vi "H3C psw cable 28G SFP+读写操作_old.vi"(6 "input_psw":u8[](array[numeric]) format="%.0x", 8 "input_data":u8[](array[numeric]) format="%.0x", 9 "input_mode":string(combo), 10 "Channel":u8 max=5 step=1, 11 "VISA":refnum<visa-resource-name>="COM6") -> (0 "A2Hequal00?":bool, 1 "result":bool, 2 "message":string, 3 "data read":u8[](array[numeric]) format="%.0x")   [LabVIEW 2011]
panel:
  out "A2h后128个字节":u8[](array[numeric]) format="%.0x"
  out "A2h前128个字节":u8[](array[numeric]) format="%.0x"
  in  "address":u8
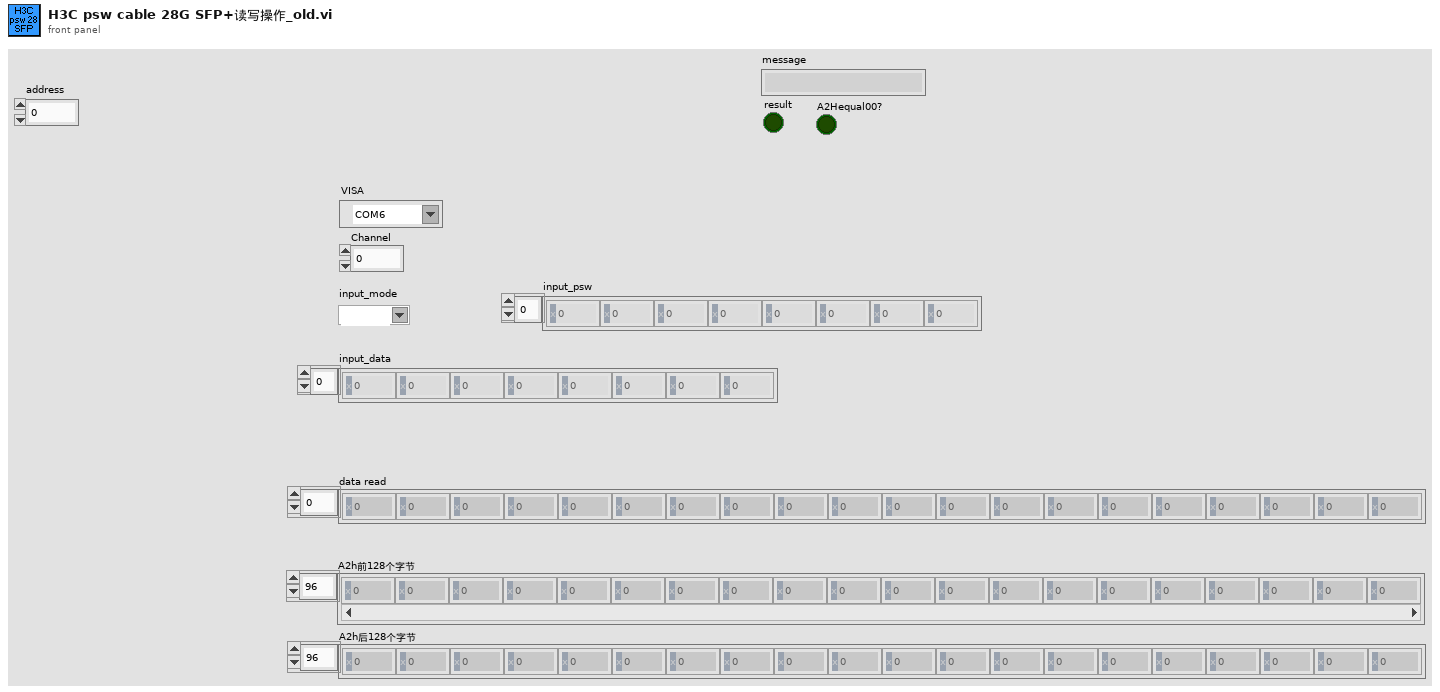
[diagram p1: front panel]
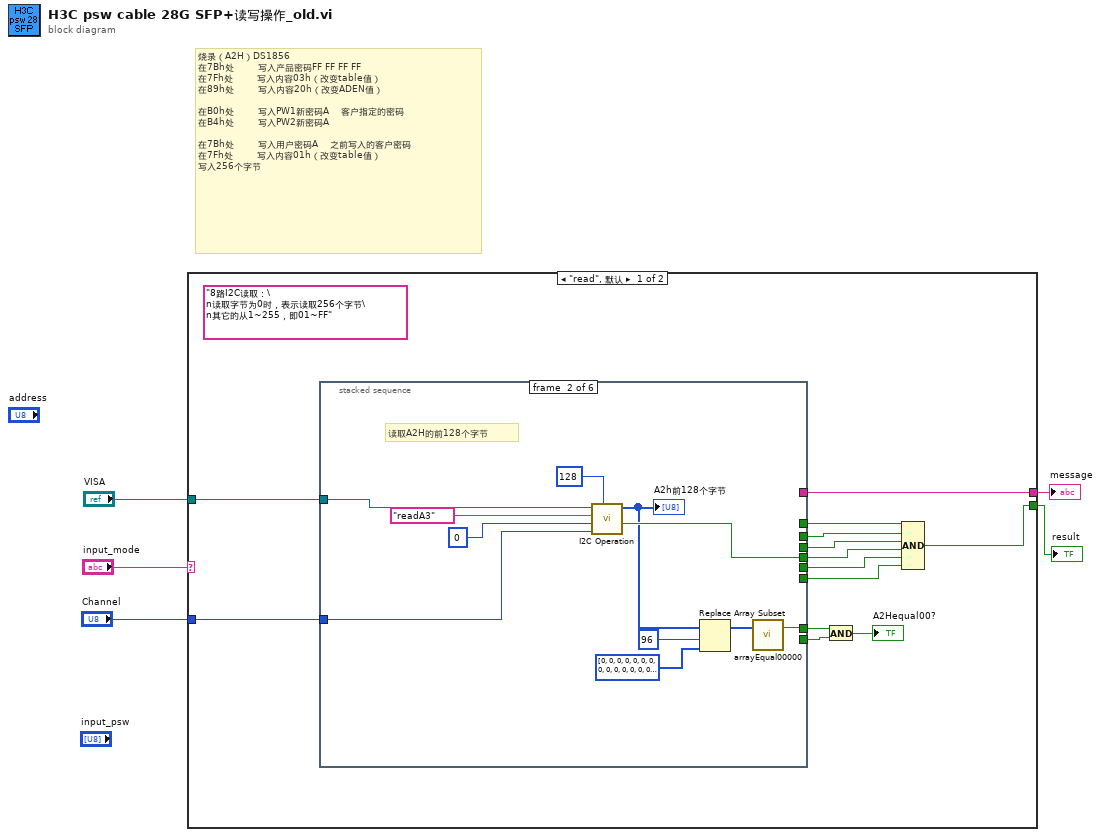
[diagram p0: block diagram]
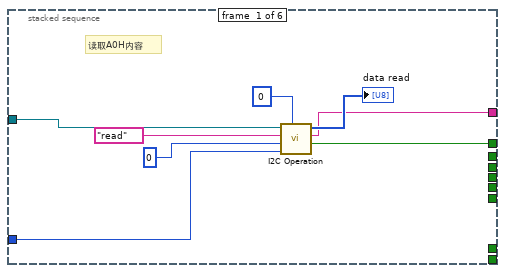
[diagram p2: hidden frame]
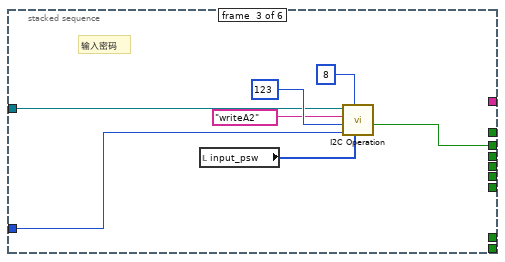
[diagram p3: hidden frame]
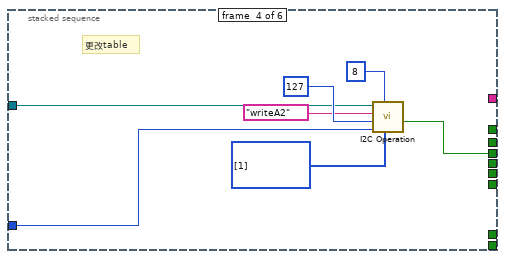
[diagram p4: hidden frame]
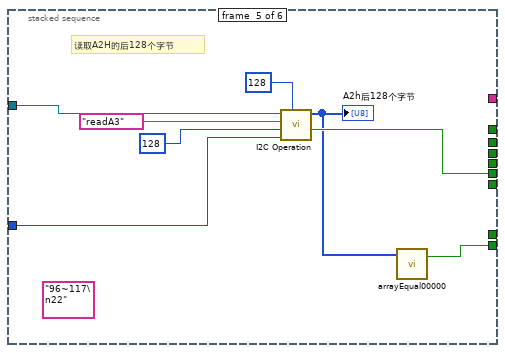
[diagram p5: hidden frame]
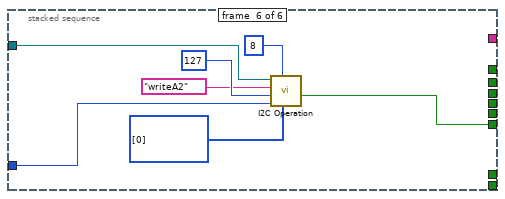
[diagram p6: hidden frame]
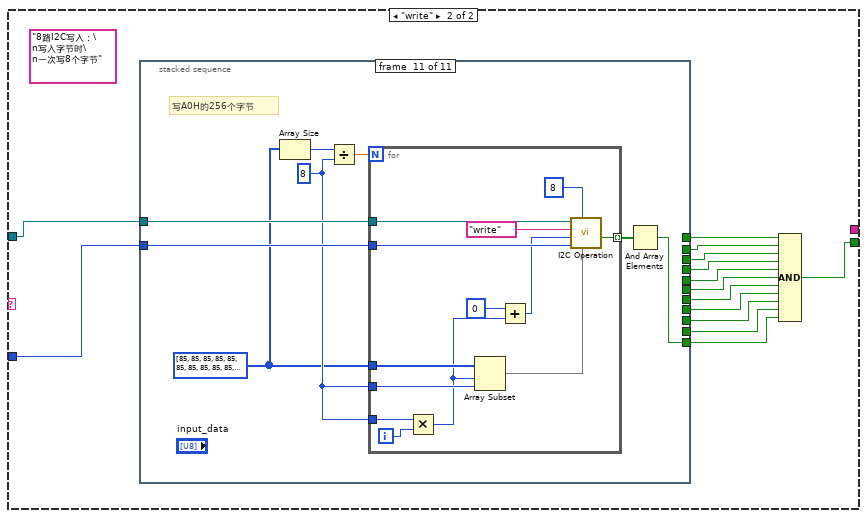
[diagram p7: hidden frame]
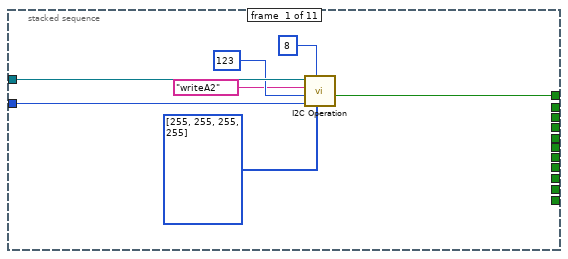
[diagram p8: hidden frame]
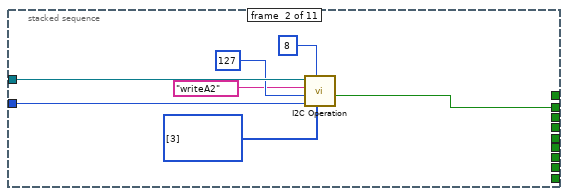
[diagram p9: hidden frame]
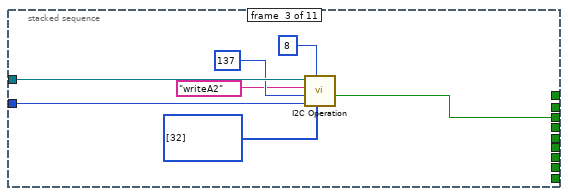
[diagram p10: hidden frame]
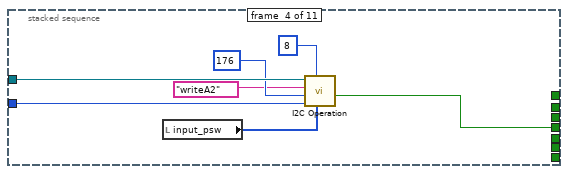
[diagram p11: hidden frame]
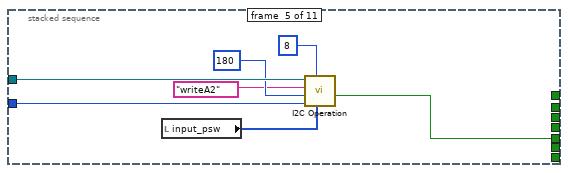
[diagram p12: hidden frame]
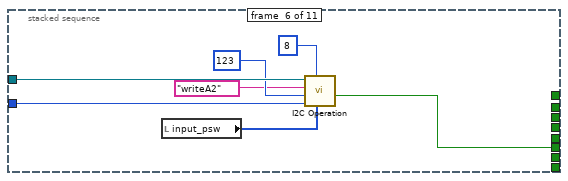
[diagram p13: hidden frame]
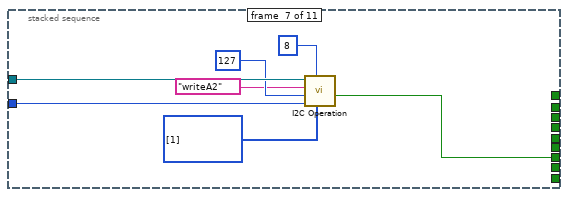
[diagram p14: hidden frame]
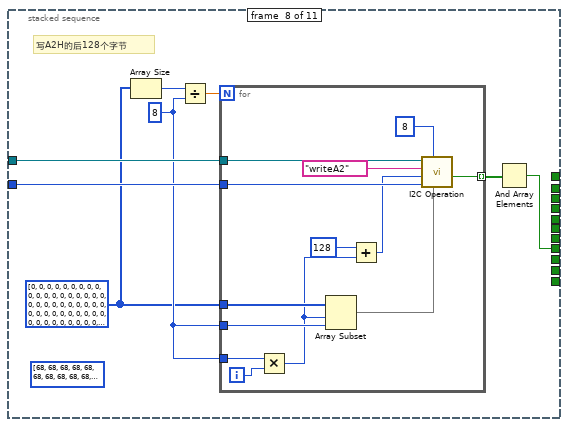
[diagram p15: hidden frame]
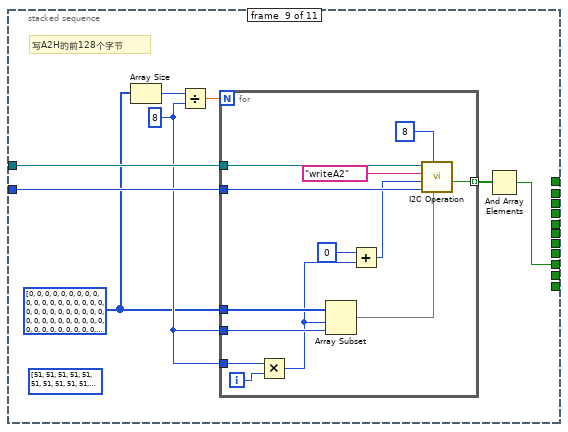
[diagram p16: hidden frame]
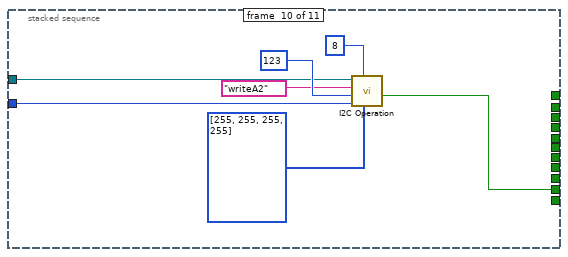
[diagram p17: hidden frame]
diagram:
  # "烧录（A2H）DS1856\n在7Bh处        写入产品密码FF FF FF FF\n在7Fh处        写入内容03h（改变table值）\n在89h处        写入内容20h（改变ADEN值）\n\n在B0h处        写入PW1新密码A    客户指定的密码\n在B4h处        写入PW2新密码A\n\n在7Bh处        写入用户密码A    之前写入的客户密码\n在7Fh处        写入内容01h（改变table值）\n写入256个字节"
  n1 = case shown="\"read\", 默认" "input_mode" {
    tunnel: "VISA" -> [w18 w80]
    tunnel: "Channel" -> [w17 w79]
    tunnel: [w16 _] -> w2
    tunnel: [w10 w67] -> w1
    frame "read", Default {
      (unwired) "8路I2C读取：\n读取字节为0时，表示读取256个字节\n其它的从1~255，即01~FF"
      n2 = stacked-sequence {
        tunnel: w18 -> [w26 w37 w40 w47 w59 w62]
        tunnel: w17 -> [w23 w34 w39 w46 w56 w61]
        tunnel: [w21 _ _ _ _ _] -> w16
        tunnel: [w20 _ _ _ _ _] -> w15
        tunnel: [_ _ w38 _ _ _] -> w14
        tunnel: [_ _ _ w45 _ _] -> w13
        tunnel: [_ w32 _ _ _ _] -> w12
        tunnel: [_ w31 _ _ _ _] -> w9
        tunnel: [_ _ _ _ w54 _] -> w11
        tunnel: [_ _ _ _ w53 _] -> w8
        tunnel: [_ _ _ _ _ w60] -> w6
        frame #0 {
          # "读取A0H内容"
          n3 = call "I2C Operation.vi"("size"=0, "Channel"=w23, "address"=u8 0, "mode"="read", "VISA"=w26) -> ("result"=w20:bool, "message"=w21:string, "Data Out"=→"data read":u8[])  [unwired: 4 in]
        }
        frame #1 {
          # "读取A2H的前128个字节"
          n4 = call "I2C Operation.vi"("size"=128, "Channel"=w34, "address"=u8 0, "mode"="readA3", "VISA"=w37) -> ("result"=w32:bool, "Data Out"=w27:u8[])  [unwired: 4 in, 1 out]
          "A2h前128个字节" <- w27
          n5 = Replace Array Subset(array=w27, new element=u8[] [0, 0, 0, 0, 0, 0, 0, 0, 0, 0, 0, 0, 0, 0, 0, 0, 0, 0, 0, 0, 0, 0], index=96 ("索引")) -> (w28:u8[])
          n6 = call "arrayEqual00000.vi"("input_array"=w28) -> ("show_bool_result"=w31:bool)  [unwired: 2 in]
        }
        frame #2 {
          # "输入密码"
          n7 = local read "input_psw"() -> (w42:u8[])
          n8 = call "I2C Operation.vi"("input_data"=w42, "size"=8, "Channel"=w39, "address"=u8 123, "mode"="writeA2", "VISA"=w40) -> ("result"=w38:bool)  [unwired: 3 in, 2 out]
        }
        frame #3 {
          # "更改table"
          n9 = call "I2C Operation.vi"("input_data"=u8[] [1], "size"=8, "Channel"=w46, "address"=u8 127, "mode"="writeA2", "VISA"=w47) -> ("result"=w45:bool)  [unwired: 3 in, 2 out]
        }
        frame #4 {
          (unwired) "96~117\n22"
          # "读取A2H的后128个字节"
          n10 = call "I2C Operation.vi"("size"=128, "Channel"=w56, "address"=u8 128, "mode"="readA3", "VISA"=w59) -> ("result"=w54:bool, "Data Out"=w52:u8[])  [unwired: 4 in, 1 out]
          "A2h后128个字节" <- w52
          n11 = call "arrayEqual00000.vi"("input_array"=w52) -> ("show_bool_result"=w53:bool)  [unwired: 2 in]
        }
        frame #5 {
          n12 = call "I2C Operation.vi"("input_data"=u8[] [0], "size"=8, "Channel"=w61, "address"=u8 127, "mode"="writeA2", "VISA"=w62) -> ("result"=w60:bool)  [unwired: 3 in, 2 out]
        }
      }
      n13 = And(x=w9, y=w8) -> (x .and. y?=→"A2Hequal00?":bool)
      n14 = Compound Arithmetic op=AND(w15, w14, w13, w12, w11, w6) -> (w10:bool)
    }
    frame "write" {
      (unwired) "8路I2C写入：\n写入字节时\n一次写8个字节"
      n15 = stacked-sequence {
        tunnel: w80 -> [w87 w94 w101 w108 w115 w122 w129 w137 w158 w175 w186]
        tunnel: w79 -> [w85 w92 w99 w106 w113 w120 w127 w136 w157 w174 w185]
        tunnel: [w81 _ _ _ _ _ _ _ _ _ _] -> w78
        tunnel: [_ w88 _ _ _ _ _ _ _ _ _] -> w77
        tunnel: [_ _ w95 _ _ _ _ _ _ _ _] -> w76
        tunnel: [_ _ _ w102 _ _ _ _ _ _ _] -> w75
        tunnel: [_ _ _ _ w109 _ _ _ _ _ _] -> w74
        tunnel: [_ _ _ _ _ w116 _ _ _ _ _] -> w73
        tunnel: [_ _ _ _ _ _ w123 _ _ _ _] -> w72
        tunnel: [_ _ _ _ _ _ _ w131 _ _ _] -> w71
        tunnel: [_ _ _ _ _ _ _ _ w152 _ _] -> w70
        tunnel: [_ _ _ _ _ _ _ _ _ w172 _] -> w69
        tunnel: [_ _ _ _ _ _ _ _ _ _ w179] -> w68
        frame #0 {
          n16 = call "I2C Operation.vi"("input_data"=u8[] [255, 255, 255, 255], "size"=8, "Channel"=w85, "address"=u8 123, "mode"="writeA2", "VISA"=w87) -> ("result"=w81:bool)  [unwired: 3 in, 2 out]
        }
        frame #1 {
          n17 = call "I2C Operation.vi"("input_data"=u8[] [3], "size"=8, "Channel"=w92, "address"=u8 127, "mode"="writeA2", "VISA"=w94) -> ("result"=w88:bool)  [unwired: 3 in, 2 out]
        }
        frame #2 {
          n18 = call "I2C Operation.vi"("input_data"=u8[] [32], "size"=8, "Channel"=w99, "address"=u8 137, "mode"="writeA2", "VISA"=w101) -> ("result"=w95:bool)  [unwired: 3 in, 2 out]
        }
        frame #3 {
          n19 = local read "input_psw"() -> (w104:u8[])
          n20 = call "I2C Operation.vi"("input_data"=w104, "size"=8, "Channel"=w106, "address"=u8 176, "mode"="writeA2", "VISA"=w108) -> ("result"=w102:bool)  [unwired: 3 in, 2 out]
        }
        frame #4 {
          n21 = local read "input_psw"() -> (w111:u8[])
          n22 = call "I2C Operation.vi"("input_data"=w111, "size"=8, "Channel"=w113, "address"=u8 180, "mode"="writeA2", "VISA"=w115) -> ("result"=w109:bool)  [unwired: 3 in, 2 out]
        }
        frame #5 {
          n23 = local read "input_psw"() -> (w118:u8[])
          n24 = call "I2C Operation.vi"("input_data"=w118, "size"=8, "Channel"=w120, "address"=u8 123, "mode"="writeA2", "VISA"=w122) -> ("result"=w116:bool)  [unwired: 3 in, 2 out]
        }
        frame #6 {
          n25 = call "I2C Operation.vi"("input_data"=u8[] [1], "size"=8, "Channel"=w127, "address"=u8 127, "mode"="writeA2", "VISA"=w129) -> ("result"=w123:bool)  [unwired: 3 in, 2 out]
        }
        frame #7 {
          (unwired) i32[] [68, 68, 68, 68, 68, 68, 68, 68, 68, 68, 68, 68, 68, 68, 68, 68, 68, 68, 68, 68, 68, 68, 68, 68, 68, 68, 68, 68, 68, 68, 68, 68, 68, 68, 68, 68, 68, 68, 68, 68, 68, 68, 68, 68, 68, 68, 68, 68, 68, 68, 68, 68, 68, 68, 68, 68, 68, 68, 68, 68, 68, 68, 68, 68, 68, 68, 68, 68, 68, 68, 68, 68, 68, 68, 68, 68, 68, 68, 68, 68, 68, 68, 68, 68, 68, 68, 68, 68, 68, 68, 68, 68, 68, 68, 68, 68, 68, 68, 68, 68, 68, 68, 68, 68, 68, 68, 68, 68, 68, 68, 68, 68, 68, 68, 68, 68, 68, 68, 68, 68, 68, 68, 68, 68, 68, 68, 68, 68]
          w133 = 8 ("y")
          w130 = u8[] [0, 0, 0, 0, 0, 0, 0, 0, 0, 0, 0, 0, 0, 0, 0, 0, 0, 0, 0, 0, 0, 0, 0, 0, 0, 0, 0, 0, 0, 0, 0, 0, 0, 0, 0, 0, 0, 0, 0, 0, 0, 0, 0, 0, 0, 0, 0, 0, 0, 0, 0, 0, 0, 0, 0, 0, 0, 0, 0, 0, 0, 0, 0, 0, 0, 0, 0, 0, 0, 0, 0, 0, 0, 0, 0, 0, 0, 0, 0, 0, 0, 0, 0, 0, 0, 0, 0, 0, 0, 0, 0, 0, 0, 0, 0, 0, 0, 0, 0, 0, 0, 0, 0, 0, 0, 0, 0, 0, 0, 0, 0, 0, 0, 0, 0, 0, 0, 0, 0, 0, 0, 0, 0, 0, 0, 0, 0, 0]
          # "写A2H的后128个字节"
          n26 = Array Size(array=w130) -> (size(s)=w135:i32)
          n27 = Divide(x=w135, y=w133) -> (x/y=w134:dbl)
          n28 = for {
            N: w134 -> [_]
            tunnel: w137 -> [w150]
            tunnel: w136 -> [w148]
            tunnel: w130 -> [w146]
            tunnel: w133 -> [w144]
            tunnel: w133 -> [w143]
            tunnel: [w138] -> w132 mode=indexing
            i -> [w145]
            n29 = Multiply(x=w144, y=w145) -> (x*y=w141:i32)
            n30 = Array Subset(array=w146, index=w141, length=w143) -> (w139:u8[])
            n31 = Add(x=u8 128 ("address"), y=w141) -> (x+y=w140:i32)
            n32 = call "I2C Operation.vi"("input_data"=w139, "size"=8, "Channel"=w148, "address"=w140, "mode"="writeA2", "VISA"=w150) -> ("result"=w138:bool)  [unwired: 3 in, 2 out]
          }
          n33 = And Array Elements(Boolean array=w132) -> (logical AND=w131:bool)
        }
        frame #8 {
          (unwired) i32[] [51, 51, 51, 51, 51, 51, 51, 51, 51, 51, 51, 51, 51, 51, 51, 51, 51, 51, 51, 51, 51, 51, 51, 51, 51, 51, 51, 51, 51, 51, 51, 51, 51, 51, 51, 51, 51, 51, 51, 51, 51, 51, 51, 51, 51, 51, 51, 51, 51, 51, 51, 51, 51, 51, 51, 51, 51, 51, 51, 51, 51, 51, 51, 51, 51, 51, 51, 51, 51, 51, 51, 51, 51, 51, 51, 51, 51, 51, 51, 51, 51, 51, 51, 51, 51, 51, 51, 51, 51, 51, 51, 51, 51, 51, 51, 51, 51, 51, 51, 51, 51, 51, 51, 51, 51, 51, 51, 51, 51, 51, 51, 51, 51, 51, 51, 51, 51, 51, 51, 51, 51, 51, 51, 51, 51, 51, 51, 51]
          w154 = 8 ("y")
          w151 = u8[] [0, 0, 0, 0, 0, 0, 0, 0, 0, 0, 0, 0, 0, 0, 0, 0, 0, 0, 0, 0, 0, 0, 0, 0, 0, 0, 0, 0, 0, 0, 0, 0, 0, 0, 0, 0, 0, 0, 0, 0, 0, 0, 0, 0, 0, 0, 0, 0, 0, 0, 0, 0, 0, 0, 0, 0, 0, 0, 0, 0, 0, 0, 0, 0, 0, 0, 0, 0, 0, 0, 0, 0, 0, 0, 0, 0, 0, 0, 0, 0, 0, 0, 0, 0, 0, 0, 0, 0, 0, 0, 0, 0, 0, 0, 0, 0, 0, 0, 0, 0, 0, 0, 0, 0, 0, 0, 0, 0, 0, 0, 0, 0, 0, 0, 0, 0, 0, 0, 0, 0, 0, 0, 0, 0, 0, 0, 0, 0]
          # "写A2H的前128个字节"
          n34 = Array Size(array=w151) -> (size(s)=w156:i32)
          n35 = Divide(x=w156, y=w154) -> (x/y=w155:dbl)
          n36 = for {
            N: w155 -> [_]
            tunnel: w158 -> [w171]
            tunnel: w157 -> [w169]
            tunnel: w151 -> [w167]
            tunnel: w154 -> [w165]
            tunnel: w154 -> [w164]
            tunnel: [w159] -> w153 mode=indexing
            i -> [w166]
            n37 = Multiply(x=w165, y=w166) -> (x*y=w162:i32)
            n38 = Array Subset(array=w167, index=w162, length=w164) -> (w160:u8[])
            n39 = Add(x=u8 0 ("address"), y=w162) -> (x+y=w161:i32)
            n40 = call "I2C Operation.vi"("input_data"=w160, "size"=8, "Channel"=w169, "address"=w161, "mode"="writeA2", "VISA"=w171) -> ("result"=w159:bool)  [unwired: 3 in, 2 out]
          }
          n41 = And Array Elements(Boolean array=w153) -> (logical AND=w152:bool)
        }
        frame #9 {
          n42 = call "I2C Operation.vi"("input_data"=u8[] [255, 255, 255, 255], "size"=8, "Channel"=w174, "address"=u8 123, "mode"="writeA2", "VISA"=w175) -> ("result"=w172:bool)  [unwired: 3 in, 2 out]
        }
        frame #10 {
          w181 = i32[] [85, 85, 85, 85, 85, 85, 85, 85, 85, 85, 85, 85, 85, 85, 85, 85, 85, 85, 85, 85, 85, 85, 85, 85, 85, 85, 85, 85, 85, 85, 85, 85, 85, 85, 85, 85, 85, 85, 85, 85, 85, 85, 85, 85, 85, 85, 85, 85, 85, 85, 85, 85, 85, 85, 85, 85, 85, 85, 85, 85, 85, 85, 85, 85, 85, 85, 85, 85, 85, 85, 85, 85, 85, 85, 85, 85, 85, 85, 85, 85, 85, 85, 85, 85, 85, 85, 85, 85, 85, 85, 85, 85, 85, 85, 85, 85, 85, 85, 85, 85, 85, 85, 85, 85, 85, 85, 85, 85, 85, 85, 85, 85, 85, 85, 85, 85, 85, 85, 85, 85, 85, 85, 85, 85, 85, 85, 85, 85, 85, 85, 85, 85, 85, 85, 85, 85, 85, 85, 85, 85, 85, 85, 85, 85, 85, 85, 85, 85, 85, 85, 85, 85, 85, 85, 85, 85, 85, 85, 85, 85, 85, 85, 85, 85, 85, 85, 85, 85, 85, 85, 85, 85, 85, 85, 85, 85, 85, 85, 85, 85, 85, 85, 85, 85, 85, 85, 85, 85, 85, 85, 85, 85, 85, 85, 85, 85, 85, 85, 85, 85, 85, 85, 85, 85, 85, 85, 85, 85, 85, 85, 85, 85, 85, 85, 85, 85, 85, 85, 85, 85, 85, 85, 85, 85, 85, 85, 85, 85, 85, 85, 85, 85, 85, 85, 85, 85, 85, 85, 85, 85, 85, 85, 85, 85, 85, 85, 85, 85, 85, 85, 85, 85, 85, 85, 85, 85]
          w182 = 8 ("y")
          # "写A0H的256个字节"
          n43 = Array Size(array=w181) -> (size(s)=w184:i32)
          n44 = Divide(x=w184, y=w182) -> (x/y=w183:dbl)
          n45 = for {
            N: w183 -> [_]
            tunnel: w186 -> [w199]
            tunnel: w185 -> [w197]
            tunnel: w181 -> [w195]
            tunnel: w182 -> [w193]
            tunnel: w182 -> [w192]
            tunnel: [w187] -> w180 mode=indexing
            i -> [w194]
            n46 = Multiply(x=w193, y=w194) -> (x*y=w190:i32)
            n47 = Array Subset(array=w195, index=w190, length=w192) -> (w188:i32[])
            n48 = Add(x=u8 0 ("address"), y=w190) -> (x+y=w189:i32)
            n49 = call "I2C Operation.vi"("input_data"=w188, "size"=8, "Channel"=w197, "address"=w189, "mode"="write", "VISA"=w199) -> ("result"=w187:bool)  [unwired: 3 in, 2 out]
          }
          n50 = And Array Elements(Boolean array=w180) -> (logical AND=w179:bool)
        }
      }
      n51 = Compound Arithmetic op=AND(w78, w77, w76, w75, w74, w73, w72, w71, w70, w69, w68) -> (w67:bool)
    }
  }
  "message" <- w2
  "result" <- w1
